vi "FXP_K_times__X_minus_Nx_times_ye__singleAxis.vi"(7 "NS":u8=5, 8 "yd_est_x":fxp<+/-,32,5>, 11 "ref(k)_x":fxp<+/-,32,5>) -> (0 "K*xerr":fxp<+/-,32,16>)   [LabVIEW 2017]
uses:
  <vilib>/Platform/TimedLoop/XDataNode/timing_clust.ctl
  <vilib>/Platform/TimedLoop/XDataNode/nitl_modes.ctl
  <vilib>/Platform/TimedLoop/XDataNode/wakeup.ctl
  typeDefs/x_vec_bram.ctl
  typeDefs/Nx_bram.ctl
  typeDefs/Kz_bram.ctl
  <vilib>/rvi/IPIntegrationNode/IPINode_Typedef/niFpgaIPINodeSupportedFamilies.ctl
  <vilib>/rvi/Emulation/niFpgaSctlEmulationGetInTimedLoop.vi
  <vilib>/rvi/Emulation/niFpgaEmulationReportErrorSimple.vi
  <vilib>/rvi/Emulation/niFpgaGetClockAttributes.vi
  <vilib>/rvi/Emulation/niFpgaCriticalErrorInLSC.vi
  <vilib>/rvi/DataTransferAndStorage/Container/Common/niFpgaContainerExecOnDevCompGetState.vi
  <vilib>/rvi/Emulation/niFpgaEmulationIsFPGAContextNoSignature.vi
  <vilib>/rvi/DataTransferAndStorage/Container/Common/niFpgaContainerGetUniqueNameForEmu.vi
  <vilib>/rvi/Emulation/niFpgaProcessEmulError.vi
  <vilib>/rvi/errors/nirviReportUnexpectedCaseInternalError (U32).vi
  <vilib>/rvi/Memory/Memory_Emulation/niFpgaMemoryEmulationCacheClearOnFirstRun.vi
  <vilib>/rvi/Memory/Memory_Emulation/nirvimemoryEmulationManagerCache_MakeExclusive.vi
  <vilib>/rvi/Memory/Memory_Emulation/niFpgaMemoryEmulationValidateCache.vi
  <vilib>/rvi/Memory/Memory_Emulation/nirvimemoryEmulationManagerCache_InsertValue.vi
  <vilib>/Utility/error.llb/Clear Errors.vi
  <vilib>/rvi/Memory/Memory_Emulation/nirvimemoryEmulationManagerCache_ReleaseExclusive.vi
  <vilib>/rvi/Memory/Memory_Emulation/nirvimemoryEmulationManagerCache_GetValue.vi
  <vilib>/rvi/Memory/Memory_Emulation/nirvimemoryEmulationManagerCache_SetValue.vi
  <vilib>/rvi/Emulation/niFpgaSctlEmulationResourceMgr.vi
  <vilib>/rvi/IPIntegrationNode/IPINode_Utilities/niFpgaIPINodeSimCore.vi
  <vilib>/Platform/TimedLoop/XDataNode/XDataNode.xnode
  <vilib>/rvi/FXPMathLib/FxpSub/XNode/nifxpmath_Sub.xnode
  <vilib>/rvi/DataTransferAndStorage/Container/XNode/niFpgaContainer.xnode
  <vilib>/rvi/Memory/Memory_Emulation/niFpgaMemoryEmulationRefIn.vi
  <vilib>/rvi/XilinxIP/XIPIN_XNode/niFpgaXIPIN.xnode
  dspAccumulators/MAC_32-15_by_32-5 1/Multiply_Accumulator_1_5751944F910F43059B315ABEE25D6FDE.dll
  <vilib>/rvi/IPIntegrationNode/IPINode_Xnode/niFpgaIPINode.xnode
  <vilib>/Platform/TimedLoop/XDataNode/XDNodeRunTimeDep.lvlib
  <vilib>/rvi/FXPMathLib/sim/FxpSim.dll
panel:
  # "|x(k)   |    -  |dcg*xss| *(r(k)-x_d(k))\n|x_u(k)|       |dcg      |\n\nx_u:  = x(k-1)\nx_d  = disturbance estimate."
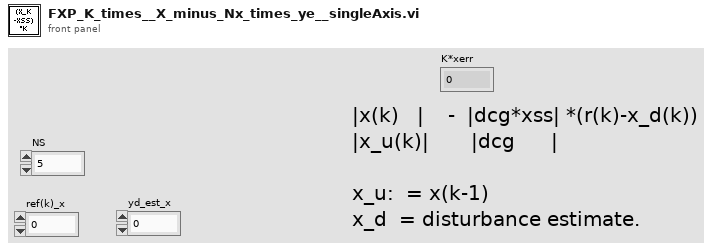
[diagram p1: front panel]
types:
  T1 = typedef "XDNodeRunTimeDep.lvlib/timing_clust.ctl" = cluster{"Expected End [f-1]":u64, "Actual End [f-1]":u64, "Finished Late? [f-1]":bool, "Expected End [i-1]":u64, "Actual End [i-1]":u64, "Finished Late? [i-1]":bool, "Expected Start [i]":u64, "Actual Start [i]":u64, "Expected Start [f]":u64, "Actual Start [f]":u64, "Source Name":string, "Structure Name":string, "Period":i64, "Deadline":i64, "Offset":i64, "Start":i64, "Priority":i32, "Timeout":i32, "Mode":T2, "Wakeup Reason":T3, "Error":errorcluster, "Source Type":string, "Secondary Source Type":string, "Global End Time":u64, "Global Start Time":u64, "Frame Duration":u64, "Iteration Duration":u64, "Assigned CPU":i32, "I/O Scan Engine Mode":u32}
  T2 = typedef "XDNodeRunTimeDep.lvlib/nitl_modes.ctl" = enum32{"No Change", "Process missed periods, maintain original phase", "Discard missed periods, maintain original phase", "Process missed periods, ignore original phase", "Discard missed periods, ignore original phase"}
  T3 = typedef "XDNodeRunTimeDep.lvlib/wakeup.ctl" = enum32{"Normal", "Aborted", "Asynchronous wakeup", "Timing source error", "Timed loop error", "Timeout"}
  T4 = typedef "Kz_bram.ctl" = refnum<k21>
  T5 = typedef "Nx_bram.ctl" = refnum<k21>
  T6 = typedef "x_vec_bram.ctl" = refnum<k21>
  T7 = typedef "niFpgaIPINodeSupportedFamilies.ctl" = cluster{"unlimited?":bool, "supported targets":string[]}
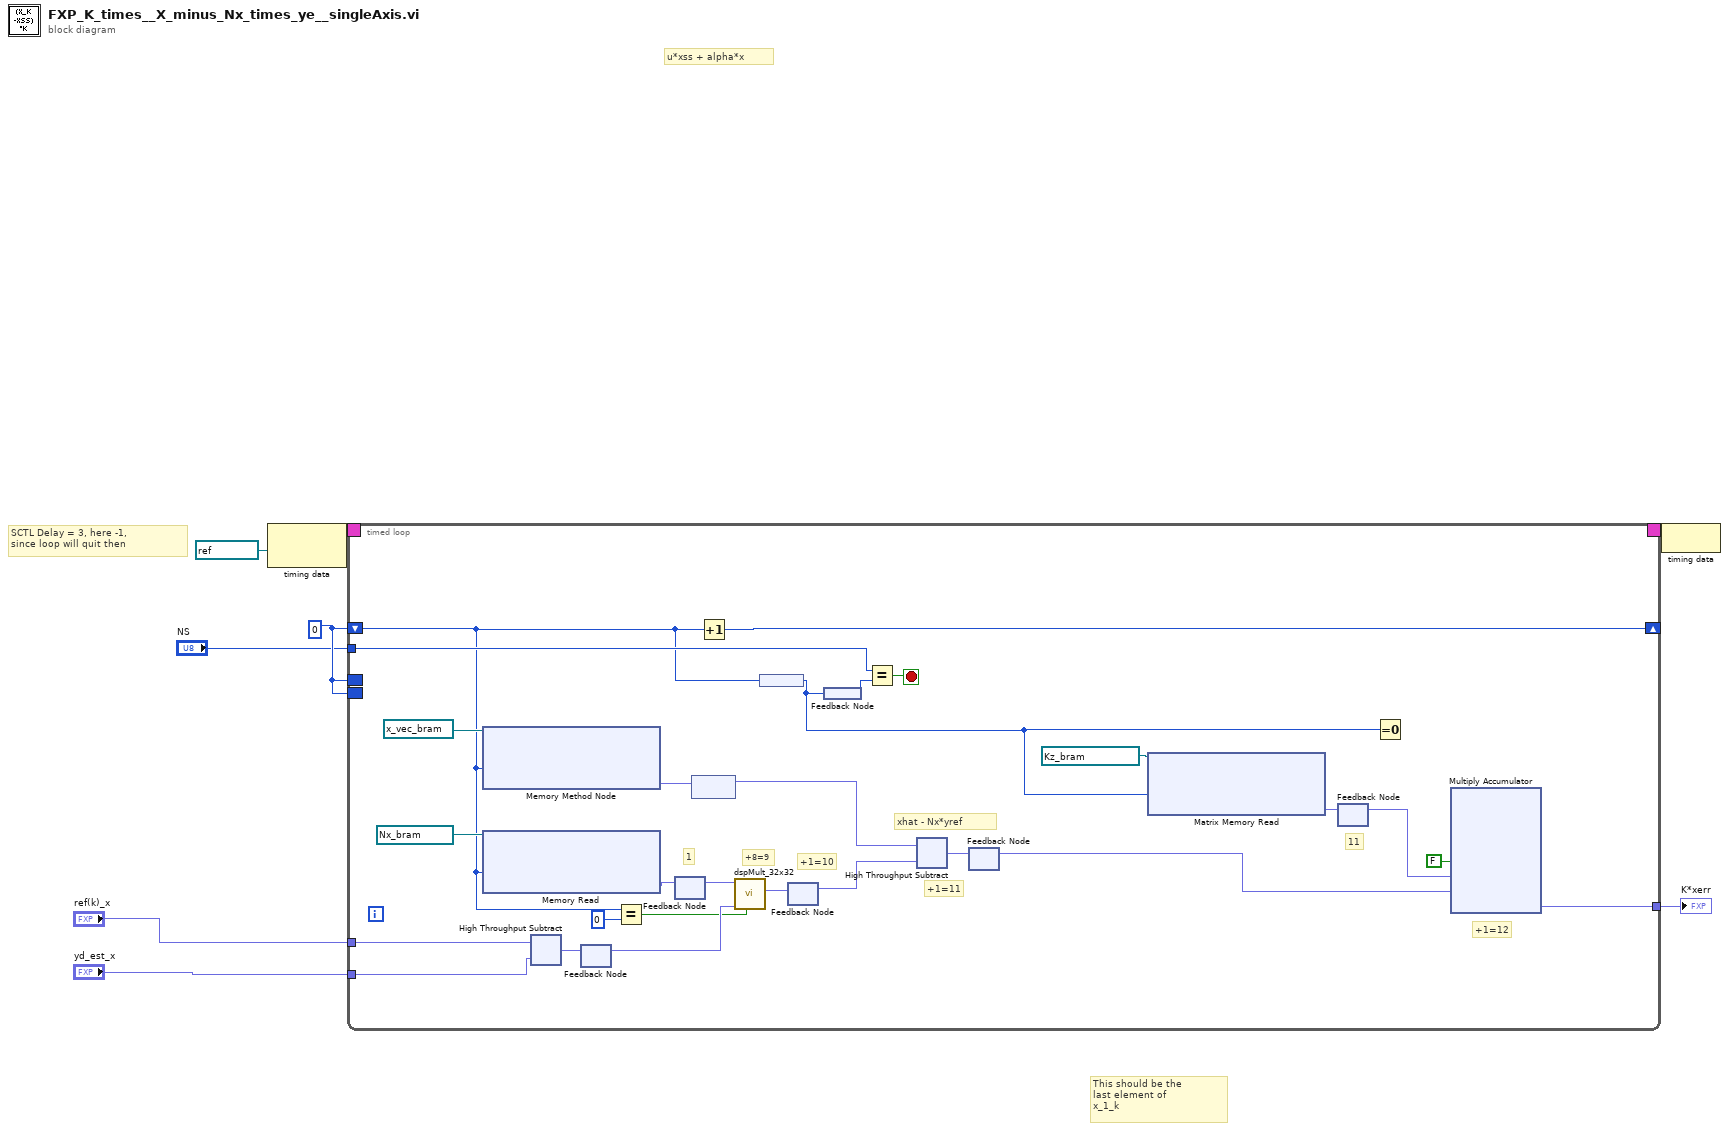
[diagram p0: block diagram]
diagram:
  w2 = u8 0
  # "This should be the \nlast element of \nx_1_k"
  # "u*xss + alpha*x"
  # "SCTL Delay = 3, here -1,\nsince loop will quit then"
  n1 = node-c288(refnum<k21> "80MHz" ("Source Name")) -> (w8:T1)
  n2 = timed-loop {
    timing: w8 -> [_]
    timing-out: [_] -> w7
    tunnel: "ref(k)_x" -> [w33]
    tunnel: "yd_est_x" -> [w32]
    shift-right: [w26] -> _
    shift-left: w2 -> [w9]
    tunnel: "NS" -> [w29]
    border: w2 -> [_]
    tunnel: [w13] -> w3
    border: w2 -> [_]
    stop <- w35 stop-if-true
    # "+1=12"
    # "11"
    # "+1=11"
    # "xhat - Nx*yref"
    # "+1=10"
    # "+8=9"
    # "1"
    n3 = xnode ("Memory Method Node")("Address"=w9, "Memory In"=T6 "xk_1_2" ("Memory")) -> ("Data"=w34:fxp<+/-,32,6>)  [unwired: 1 out]
    n4 = xnode ("Memory Read")("Address"=w9, "Memory In"=T5 "Nx_col1" ("Nx")) -> ("Data"=w31:fxp<+/-,32,2>)  [unwired: 1 out]
    n5 = xnode "High Throughput Subtract"("x"=w33, "y"=w32) -> ("x-y"=w30:fxp<+/-,32,5>)
    n6 = feedback #1() -> (w25:fxp<+/-,32,5>)  [unwired: 1 in]
    n7 = feedback-in #1(w30) -> ()
    n8 = Equal?(x=w9, y=u8 0) -> (x = y?=w23:bool)
    n9 = feedback #2() -> (w27:fxp<+/-,32,2>)  [unwired: 1 in]
    n10 = feedback-in #2(w31) -> ()
    n11 = feedback #3() -> (w22:fxp<+/-,32,6>)  [unwired: 1 in]
    n12 = feedback-in #3(w34) -> ()
    n13 = Increment(x=w9) -> (x+1=w26:u8)
    n14 = call "dspMult_32x32.vi"("sclr"=w23, "b"=w25, "a"=w27) -> ("p"=w28:fxp<+/-,64,10>)  [unwired: 8 in]
    n15 = feedback #4() -> (w11:u8)
    n16 = feedback-in #4(w9) -> ()
    n17 = feedback #5() -> (w21:fxp<+/-,64,10>)  [unwired: 1 in]
    n18 = feedback-in #5(w28) -> ()
    n19 = feedback #6() -> (w12:u8)
    n20 = feedback-in #6(w11) -> ()
    n21 = Equal?(x=w29, y=w12) -> (x = y?=w35:bool)
    n22 = xnode "High Throughput Subtract"("x"=w22, "y"=w21) -> ("x-y"=w14:fxp<+/-,32,6>)
    n23 = feedback #7() -> (w15:fxp<+/-,32,6>)  [unwired: 1 in]
    n24 = feedback-in #7(w14) -> ()
    n25 = xnode "Matrix Memory Read"("Address"=w11, "Memory In"=T4 "K_FXP_row1" ("Memory")) -> ("Data"=w17:fxp<+/-,32,10>)  [unwired: 1 out]
    n26 = feedback #8() -> (w16:fxp<+/-,32,10>)  [unwired: 1 in]
    n27 = feedback-in #8(w17) -> ()
    n28 = Equal To 0?(x=w11) -> ()  [unwired: 1 out]
    n29 = xnode ("Multiply Accumulator")("sclr"=FALSE, "a"=w16, "b"=w15) -> ("s"=w13:fxp<+/-,32,16>)  [unwired: 2 in]
  }
  "K*xerr" <- w3
  n30 = node-c288(w7) -> ()
